vi "De Initialization.vi"(8 "Error In":errorcluster, 9 "Intialize?":bool=TRUE, 10 "Inputs":T1, 11 "Start SM":dbl=10.0 format="%#_13g") -> (0 "error out":errorcluster, 1 "Completed":bool, 3 "Results":cluster{"Pinch Force":dbl}, 4 "Status":cluster{"Status":string, "Elapsed Time":dbl}, 5 "Graph":dbl[][](array[numeric]))   [LabVIEW 2017]
doc: "Changelog:\n\n------------\nv0.1:\n- Bypass sensor 1 for all front\n\nv0.1:\n- Start Travel time taken from when the start moving command is given (previous state)\n- Total travel time is taken until the movement is stopped"
uses:
  controls/Model Name.ctl
  controls/All Inputs.ctl
  controls/SACB DI.ctl
  controls/De Intialization.ctl
  controls/FGV DO.ctl
panel:
  in  "Model Name":T3
  in  "minimum change 3":dbl=1.0 format="%#_13g"
  in  "minimum change 2":dbl=1.0 format="%#_13g"
  in  "minimum change":dbl=1.0 format="%#_13g"
  in  "AutoCommand":u32=30
  in  "Stall Time":u32=200
  out "Waveform Graph":dbl[][](graph)
  in  "Delay (for Rest)":u32=500
  in  "Timeout (ms)":u32=15000
  # "Inputs"
  # "Variables"
  # "Outputs"
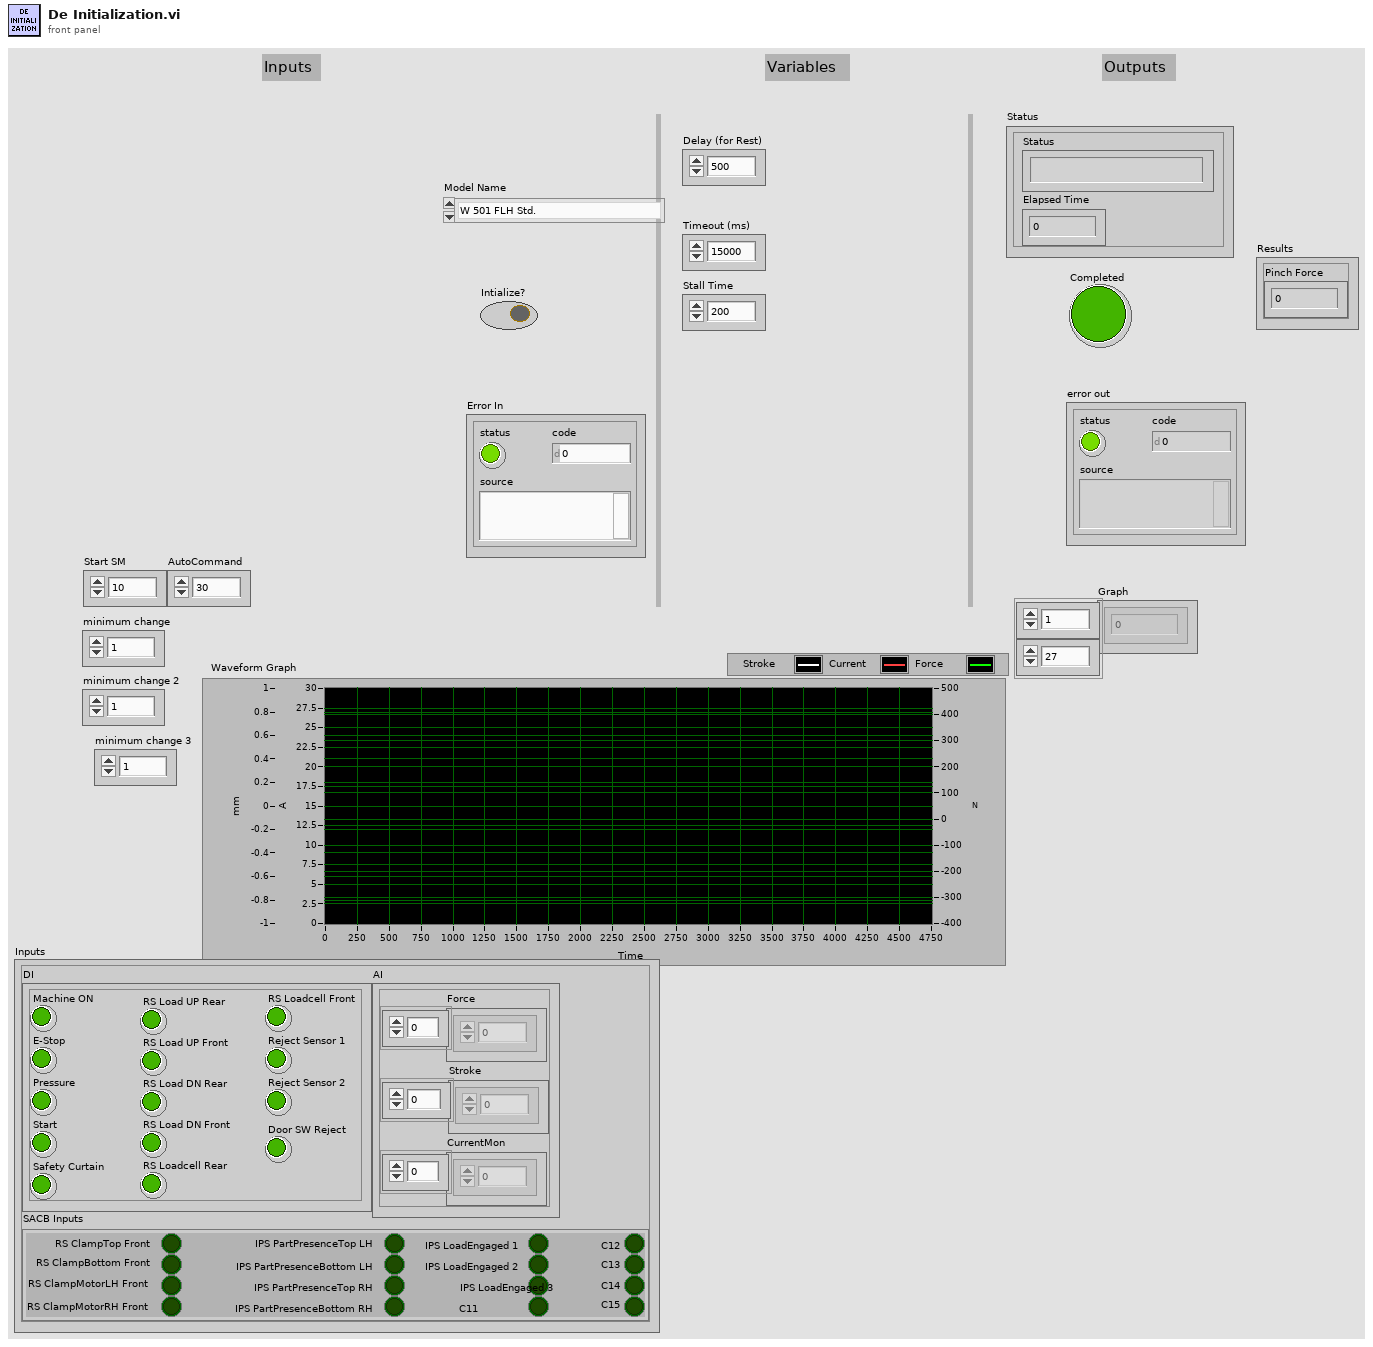
[diagram p1: front panel]
types:
  T1 = typedef "All Inputs.ctl" = cluster{"DI":cluster{"Machine ON":bool, "E-Stop":bool, "Pressure":bool, "Start":bool, "Safety Curtain":bool, "RS Load UP Rear":bool, "RS Load UP Front":bool, "RS Load DN Rear":bool, "RS Load DN Front":bool, "RS Loadcell Rear":bool, "RS Loadcell Front":bool, "Reject Sensor 1":bool, "Reject Sensor 2":bool, "Door SW Reject":bool}, "AI":cluster{"Force":dbl[], "Stroke":dbl[], "CurrentMon":dbl[]}, "SACB Inputs":T2}
  T2 = typedef "SACB DI.ctl" = cluster{"RS ClampTop Front":bool, "RS ClampBottom Front":bool, "RS ClampMotorLH Front":bool, "RS ClampMotorRH Front":bool, "IPS PartPresenceTop LH":bool, "IPS PartPresenceBottom LH":bool, "IPS PartPresenceTop RH":bool, "IPS PartPresenceBottom RH":bool, "IPS LoadEngaged 1":bool, "IPS LoadEngaged 2":bool, "IPS LoadEngaged 3":bool, "C11":bool, "C12":bool, "C13":bool, "C14":bool, "C15":bool}
  T3 = typedef "Model Name.ctl" = enum16{"W 501 FLH Std.", "W 501 FRH Std.", "W 601 FR RH Std", "W 601 FR LH Std", "W 601 RR RH Std", "W 601 RR LH Std", "W 601 FR RH AP", "W 601 FR LH AP", "W 601 RR RH AP", "W 601 RR LH AP"}
  T4 = typedef "De Intialization.ctl" = enum16{"Initialize", "Check Bottom Position", "Go Down", "Wait for Stall", "Go Up", "Wait for Top Stall", "Manual UP-1", "Manual UP-2", "Initialize Counter", "Auto UP-1", "Auto UP-2", "Wait for Stop", "Done", "Error"}
  T5 = typedef "FGV DO.ctl" = enum16{"Initialize", "Start Task", "Clamping", "Load CYL", "Contactors", "Loadcell CYL", "BSL", "Read DO", "Clear Tasks", "Clear Task"}
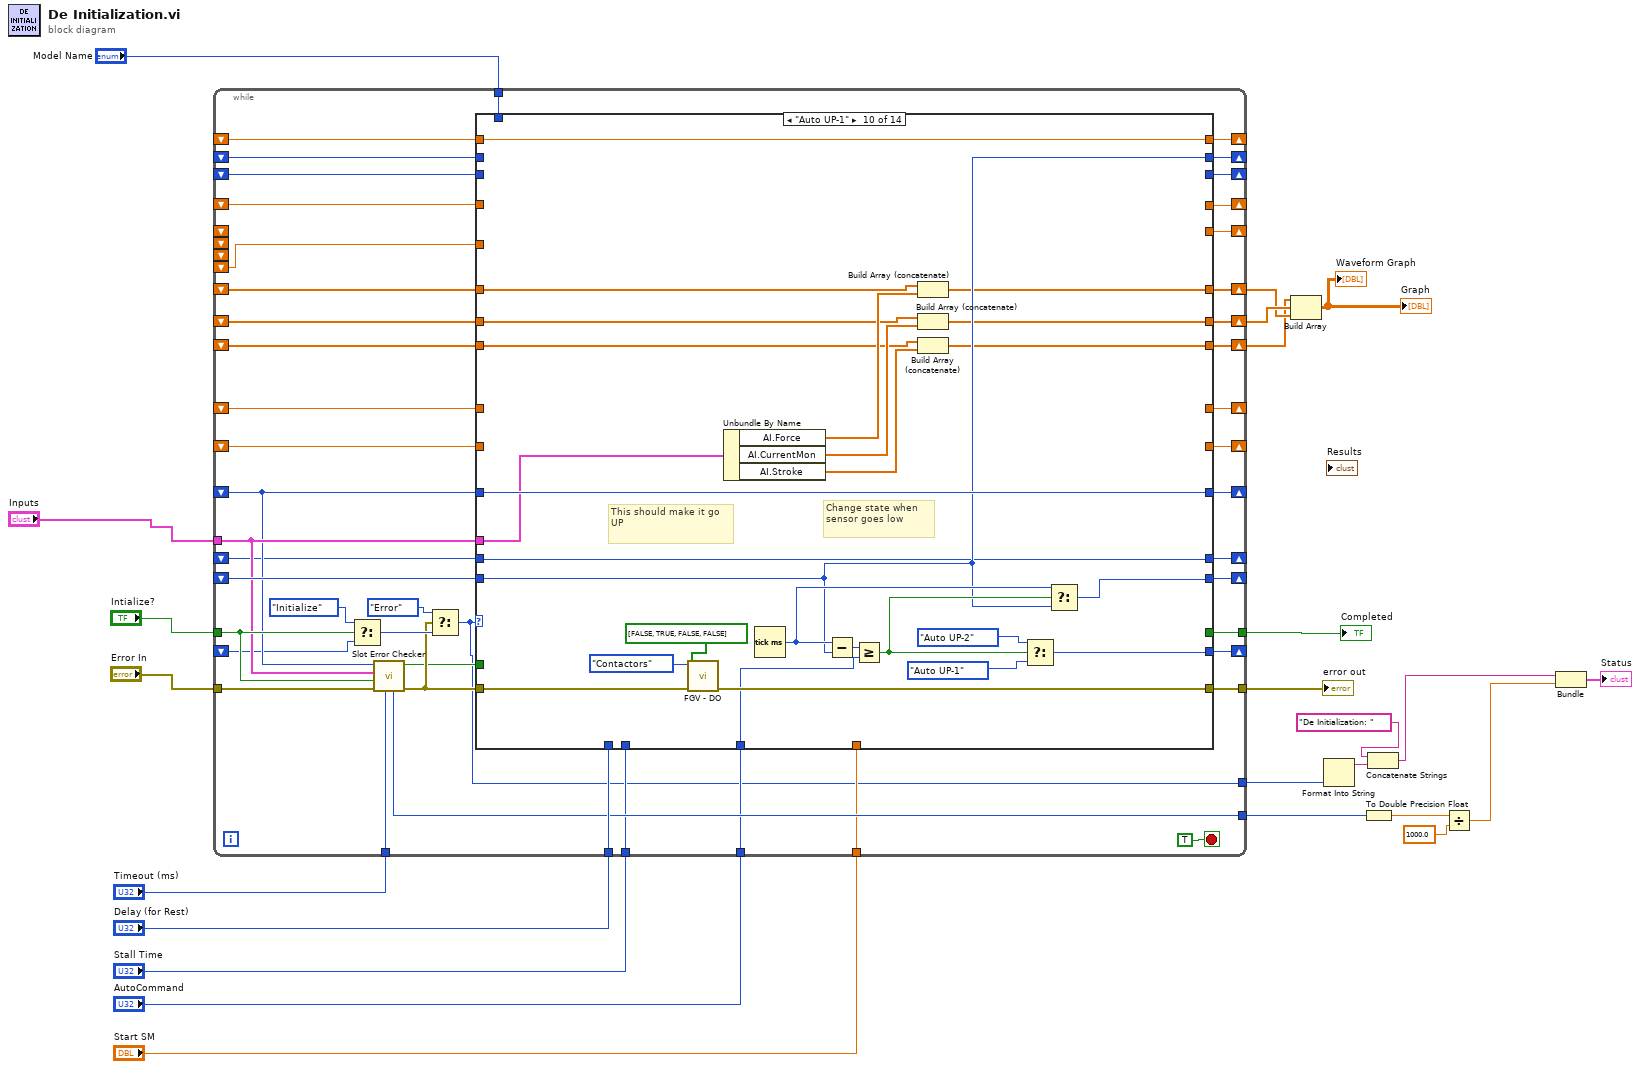
[diagram p0: block diagram]
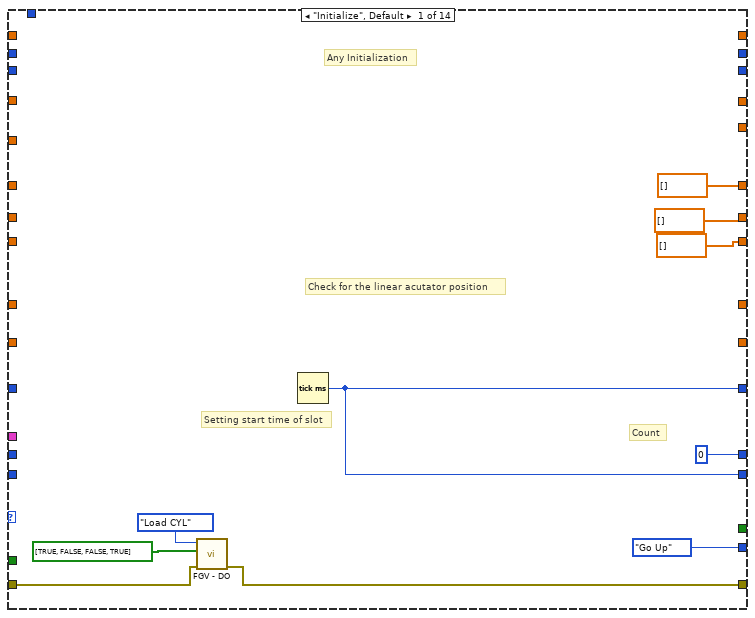
[diagram p2: hidden frame]
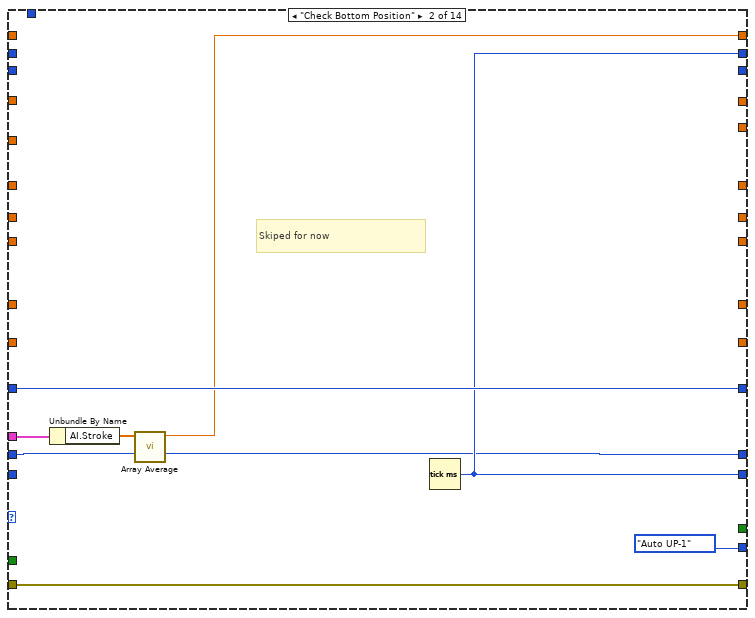
[diagram p3: hidden frame]
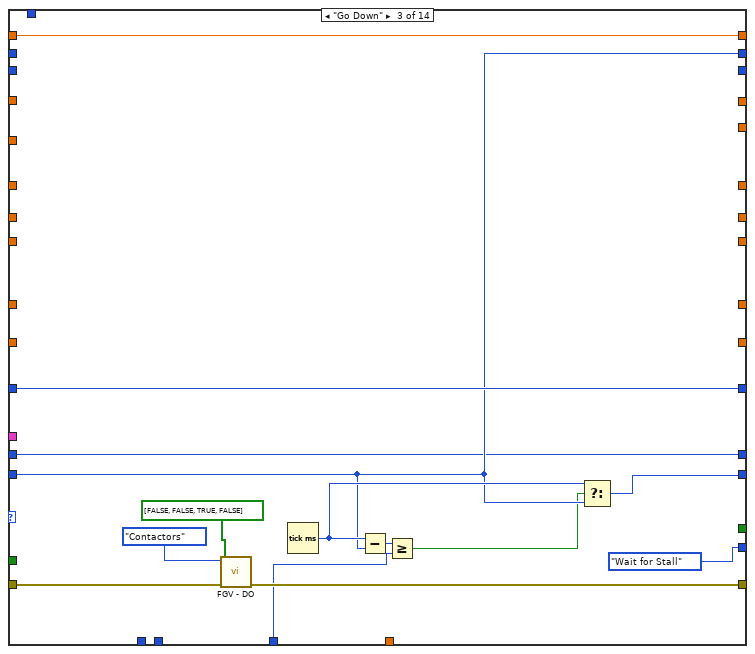
[diagram p4: hidden frame]
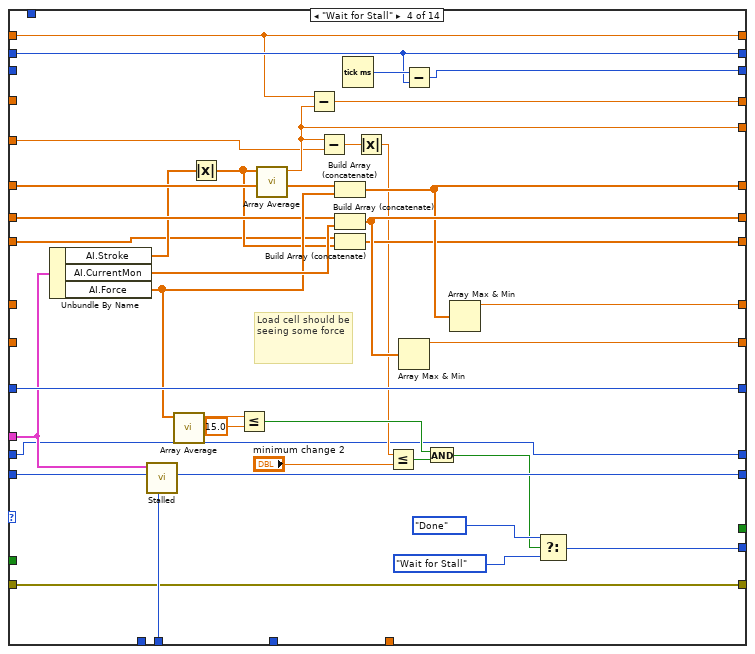
[diagram p5: hidden frame]
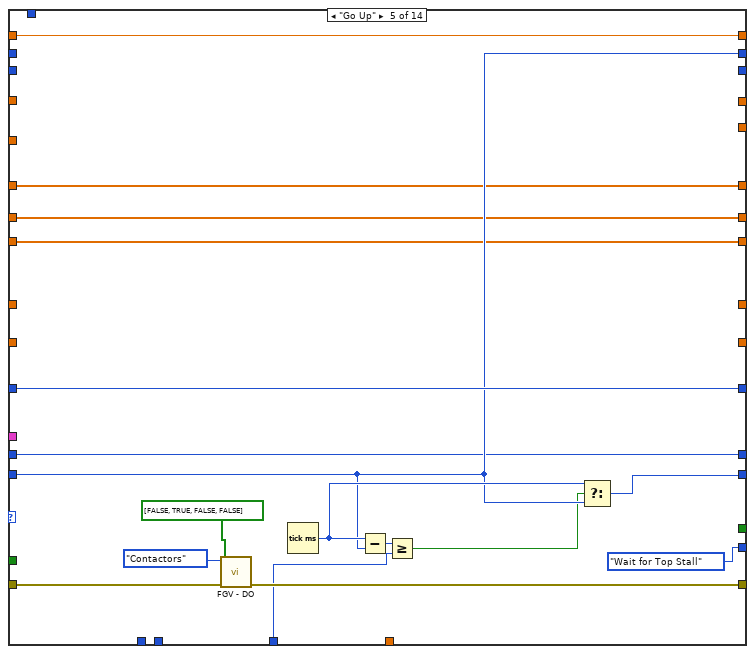
[diagram p6: hidden frame]
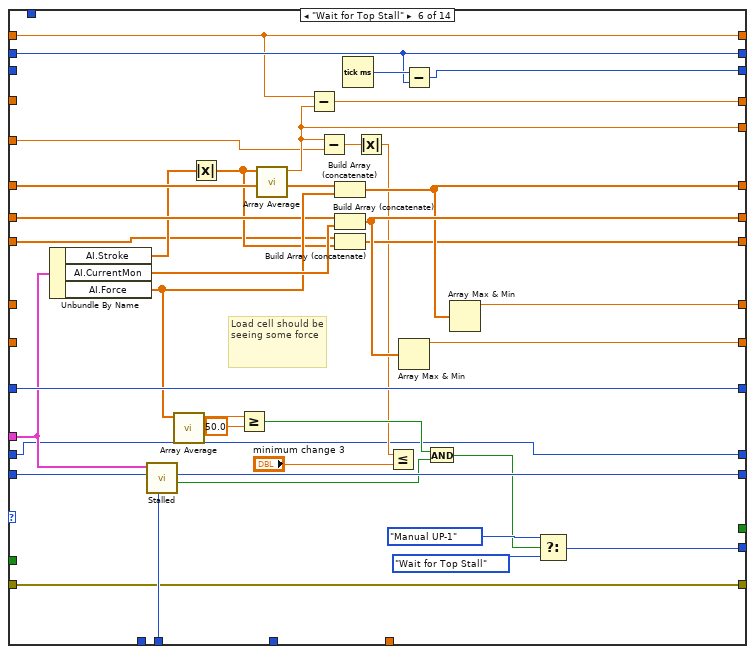
[diagram p7: hidden frame]
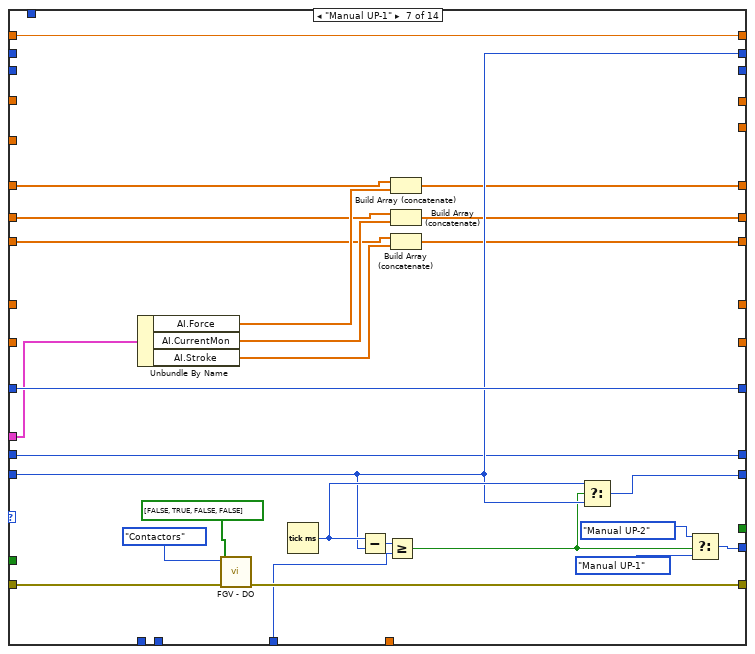
[diagram p8: hidden frame]
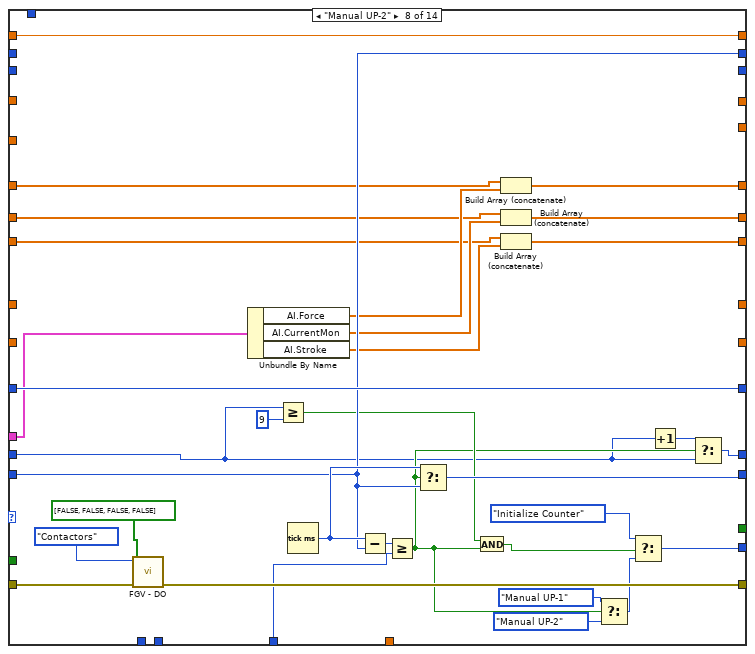
[diagram p9: hidden frame]
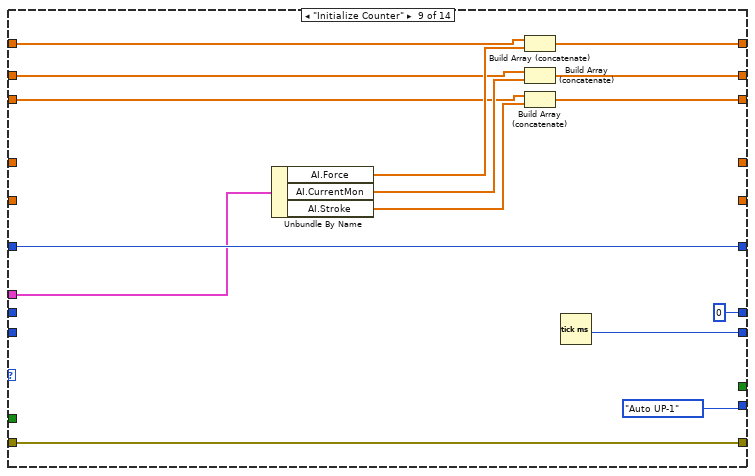
[diagram p10: hidden frame]
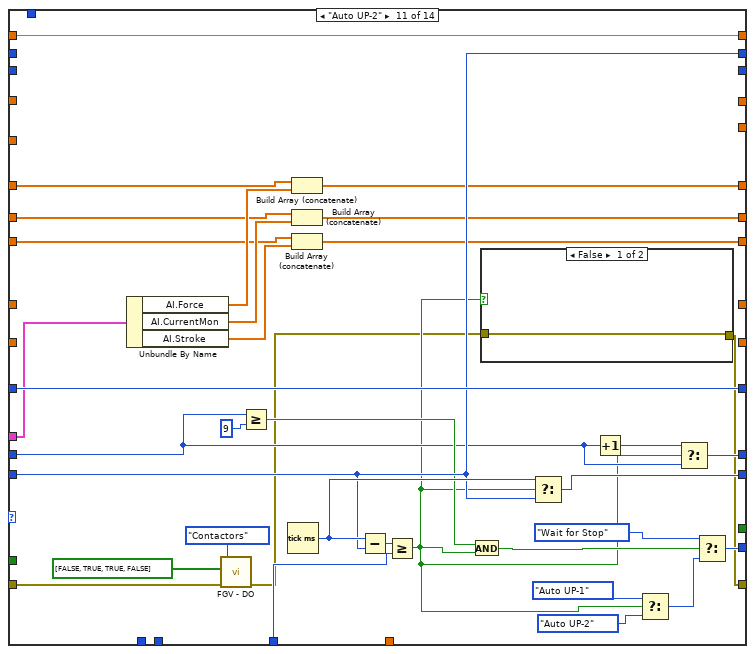
[diagram p11: hidden frame]
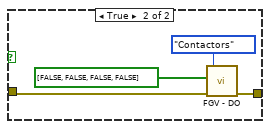
[diagram p12: hidden frame]
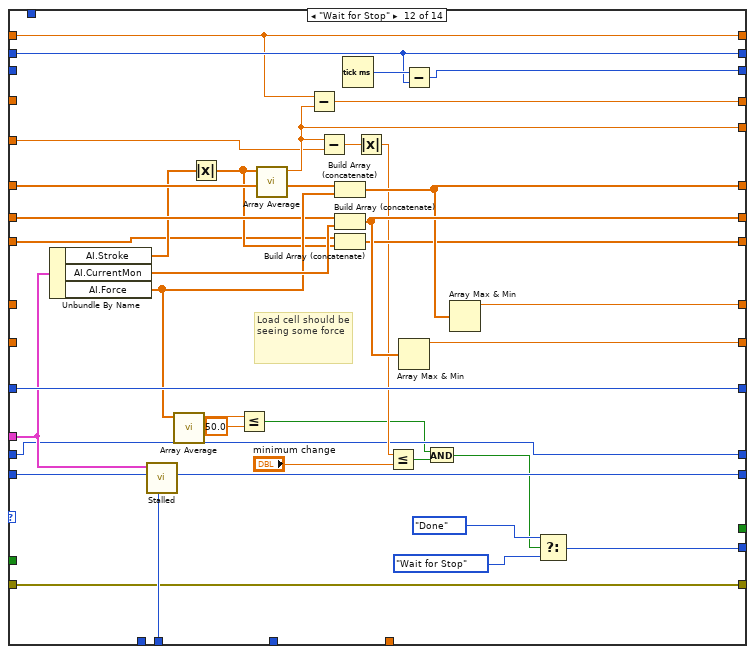
[diagram p13: hidden frame]
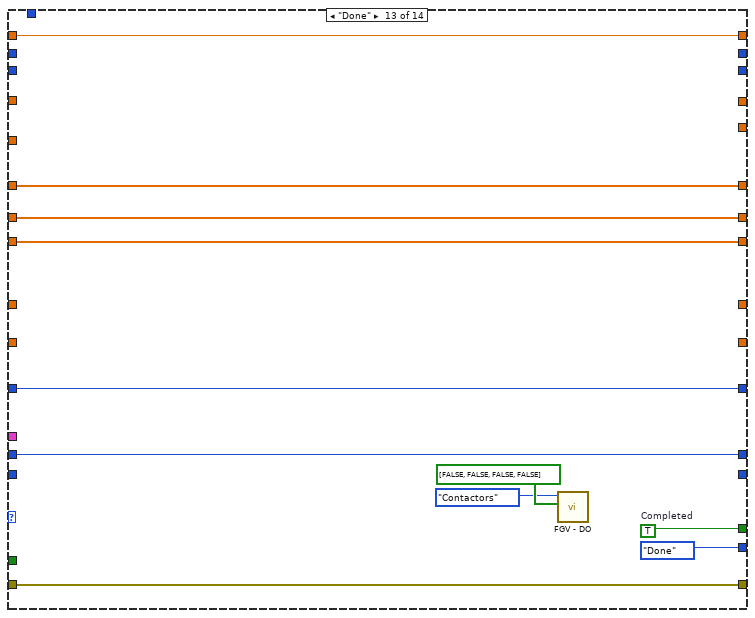
[diagram p14: hidden frame]
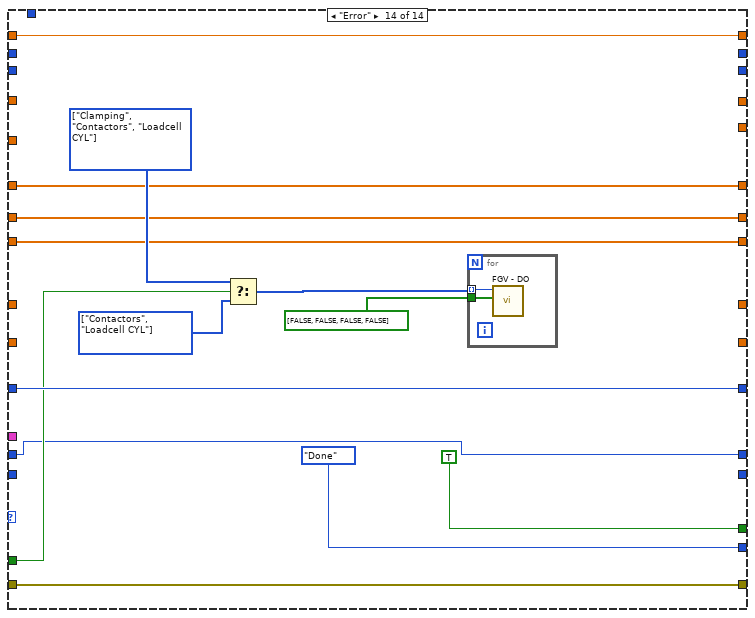
[diagram p15: hidden frame]
diagram:
  n1 = while {
    tunnel: "Intialize?" -> [w62]
    shift-right: [w69] -> _
    shift-left: _ -> [w26]
    shift-right: [w68] -> _
    shift-left: _ -> [w67]
    tunnel: "Error In" -> [w63]
    tunnel: [w66] -> w24
    tunnel: [w65] -> w23
    tunnel: "Inputs" -> [w61]
    shift-right: [w64] -> _
    shift-left: _ -> [w60]
    tunnel: "Delay (for Rest)" -> [w56]
    tunnel: "Timeout (ms)" -> [w55]
    tunnel: "Model Name" -> [w54]
    shift-right: [w53] -> _
    shift-left: _ -> [w52]
    shift-right: [w51] -> w7
    shift-left: _ -> [w50]
    shift-right: [w49] -> _
    shift-left: _ -> [w48]
    shift-right: [w47] -> _
    shift-left: _ -> [w46]
    tunnel: [w45] -> w14
    shift-right: [w44] -> _
    shift-left: _ -> [w43]
    shift-right: [w42] -> w13
    shift-left: _ -> [w41]
    shift-right: [w40] -> w11
    shift-left: _ -> [w39]
    shift-right: [w38] -> _
    shift-left: _ -> [w37]
    shift-right: [w36] -> _
    shift-left: _ -> [w35]
    tunnel: "Stall Time" -> [w34]
    tunnel: "Start SM" -> [w32]
    tunnel: "AutoCommand" -> [w31]
    shift-right: [w30] -> _
    shift-left: _ -> [_]
    shift-left: _ -> [_]
    shift-left: _ -> [_]
    shift-left: _ -> [w29]
    shift-right: [w28] -> _
    shift-left: _ -> [w27]
    tunnel: [w25] -> w1
    stop <- TRUE stop-if-true
    n2 = Select(t=De_Intialization."Initialize", s=w62, f=w26) -> (s? t:f=w59:T4)
    n3 = call "Slot Error Checker.vi"("Timeout (ms)"=w55, "error in (no error)"=w63, "Intialize?"=w62, "Inputs"=w61, "start time"=w60) -> ("error out"=w58:errorcluster, "Safety Interrupt?"=w33:bool, "Slot Time"=w45:u32)  [unwired: 4 in]
    n4 = Select(t=De_Intialization."Error", s=w58, f=w59) -> (s? t:f=w25:T4)
    n5 = case shown="\"Auto UP-1\"" w25 {
      tunnel: [De_Intialization."Go Up" De_Intialization."Auto UP-1" De_Intialization."Wait for Stall" w136 De_Intialization."Wait for Top Stall" w190 w213 w247 De_Intialization."Auto UP-1" w287 w322 w366 De_Intialization."Done" De_Intialization."Done"] -> w69
      tunnel: [w81 w83 w94 w127 w148 w181 w209 w243 w264 w282 w318 w357 _ _] -> w68
      tunnel: w67 -> [_ _ w95 w139 w149 w193 w210 w244 _ w283 w319 w369 _ _]
      tunnel: w58 -> [w78 w88 w93 w116 w147 w170 w207 w241 w265 w280 w328 w346 w380 w395]
      tunnel: [w77 w88 w103 w116 w157 w170 w220 w253 w265 w294 w305 w346 w380 w395] -> w66
      tunnel: [_ _ _ _ _ _ _ _ _ _ _ _ w379 TRUE ("Completed")] -> w65
      tunnel: w61 -> [_ w85 _ w105 _ w160 w204 w227 w254 w269 w295 w336 _ _]
      tunnel: [w81 w89 w101 w140 w155 w194 w218 w251 w267 w292 w326 w370 w378 w392] -> w64
      tunnel: w60 -> [_ w89 w101 w140 w155 w194 w218 w251 w267 w292 w326 w370 w378 w392]
      tunnel: w56 -> [_ _ _ _ _ _ _ _ _ _ _ _ _ _]
      tunnel: w54 -> [_ _ _ _ _ _ _ _ _ _ _ _ _ _]
      tunnel: [_ w83 w95 w126 w149 w180 w210 w244 _ w283 w319 w356 _ _] -> w53
      tunnel: w52 -> [_ _ _ w126 _ w180 _ _ _ _ _ w356 _ _]
      tunnel: [dbl[] [] _ _ w128 w141 w182 w196 w221 w257 w270 w296 w358 w377 w385] -> w51
      tunnel: w50 -> [_ _ _ w106 w141 w161 w197 w224 w258 w271 w297 w337 w377 w385]
      tunnel: [_ _ _ w129 _ w183 _ _ _ _ _ w359 _ _] -> w49
      tunnel: w48 -> [_ _ _ _ _ _ _ _ _ _ _ _ _ _]
      tunnel: [_ _ _ w134 _ w188 _ _ _ _ _ w364 _ _] -> w47
      tunnel: w46 -> [_ _ _ _ _ _ _ _ _ _ _ _ _ _]
      tunnel: [_ w84 w100 w117 w154 w171 w217 w250 _ w291 w325 w347 w375 w391] -> w44
      tunnel: w43 -> [_ _ w100 w117 w154 w171 w217 w250 _ w291 w325 w347 w375 w391]
      tunnel: [dbl[] [] _ _ w132 w142 w186 w199 w223 w256 w272 w298 w362 w376 w384] -> w42
      tunnel: w41 -> [_ _ _ w122 w142 w176 w200 w225 w259 w273 w299 w352 w376 w384]
      tunnel: [dbl[] [] _ _ w131 w143 w185 w201 w222 w255 w274 w300 w361 w372 w383] -> w40
      tunnel: w39 -> [_ _ _ w121 w143 w175 w202 w226 w260 w275 w301 w351 w372 w383]
      tunnel: [_ _ _ w130 _ w184 _ _ _ _ _ w360 _ _] -> w38
      tunnel: w37 -> [_ _ _ _ _ _ _ _ _ _ _ _ _ _]
      tunnel: [_ _ _ w114 _ w168 _ _ _ _ _ w345 _ _] -> w36
      tunnel: w35 -> [_ _ _ _ _ _ _ _ _ _ _ _ _ _]
      tunnel: w34 -> [_ _ _ w120 _ w174 _ _ _ _ _ w350 _ _]
      tunnel: w33 -> [_ _ _ _ _ _ _ _ _ _ _ _ _ w386]
      tunnel: w32 -> [_ _ _ _ _ _ _ _ _ _ _ _ _ _]
      tunnel: w31 -> [_ _ w97 _ w151 _ w212 w246 _ w286 w321 _ _ _]
      tunnel: [_ _ _ w113 _ w167 _ _ _ _ _ w344 _ _] -> w30
      tunnel: w29 -> [_ _ _ w112 _ w166 _ _ _ _ _ w343 _ _]
      tunnel: [0 w82 w91 w104 w145 w159 w205 w239 0 w279 w316 w335 w371 w382] -> w28
      tunnel: w27 -> [_ w82 w91 w104 w145 w159 w205 w231 _ w279 w308 w335 w371 w382]
      frame "Initialize", Default {
        # "Check for the linear acutator position"
        # "Count"
        # "Setting start time of slot"
        # "Any Initialization"
        n6 = call "FGV - DO.vi"("error in"=w78, "Digital Outs"=bool[] [TRUE, FALSE, FALSE, TRUE], "State"=FGV_DO."Load CYL") -> ("error out"=w77:errorcluster)  [unwired: 7 in, 1 out]
        n7 = Tick Count (ms)() -> (millisecond timer value=w81:u32)
      }
      frame "Check Bottom Position" {
        # "Skiped for now"
        n8 = Unbundle By Name(w85) -> ("AI.Stroke"=w86:dbl[])
        n9 = call "Array Average.vi"("data"=w86) -> ("Numeric"=w84:dbl)  [unwired: 10 in]
        n10 = Tick Count (ms)() -> (millisecond timer value=w83:u32)
      }
      frame "Go Down" {
        n11 = call "FGV - DO.vi"("error in"=w93, "Digital Outs"=bool[] [FALSE, FALSE, TRUE, FALSE], "State"=FGV_DO."Contactors") -> ("error out"=w103:errorcluster)  [unwired: 7 in, 1 out]
        n12 = Tick Count (ms)() -> (millisecond timer value=w96:u32)
        n13 = Subtract(x=w96, y=w95) -> (x-y=w98:u32)
        n14 = Greater Or Equal?(x=w98, y=w97) -> (x >= y?=w92:bool)
        n15 = Select(t=w96, s=w92, f=w95) -> (s? t:f=w94:u32)
      }
      frame "Wait for Stall" {
        # "Load cell should be seeing some force"
        n16 = Unbundle By Name(w105) -> ("AI.Stroke"=w119:dbl[], "AI.CurrentMon"=w133:dbl[], "AI.Force"=w124:dbl[])
        n17 = call "Stalled.vi"("Stall Time (ms)"=w120, "millisecond timer value in"=w139, "Inputs"=w105) -> ("millisecond timer value out"=w127:u32)  [unwired: 7 in, 1 out]
        n18 = call "Array Average.vi"("data"=w124) -> ("Numeric"=w123:dbl)  [unwired: 10 in]
        n19 = Absolute Value(x=w119) -> (abs(x)=w118:dbl[])
        n20 = Less Or Equal?(x=w123, y=15.0) -> (x <= y?=w115:bool)
        n21 = call "Array Average.vi"("data"=w118) -> ("Numeric"=w113:dbl)  [unwired: 10 in]
        n22 = Subtract(x=w117, y=w113) -> (x-y=w114:dbl)
        n23 = Subtract(x=w113, y=w112) -> (x-y=w111:dbl)
        n24 = Build Array (concatenate)(w121, w124) -> (w131:dbl[])
        n25 = Build Array (concatenate)(w122, w133) -> (w132:dbl[])
        n26 = Build Array (concatenate)(w106, w118) -> (w128:dbl[])
        n27 = Tick Count (ms)() -> (millisecond timer value=w135:u32)
        n28 = Absolute Value(x=w111) -> (abs(x)=w110:dbl)
        n29 = Less Or Equal?(x=w110, y="minimum change 2") -> (x <= y?=w107:bool)
        n30 = Array Max & Min(array=w132) -> (max value=w134:dbl)  [unwired: 3 out]
        n31 = Subtract(x=w135, y=w126) -> (x-y=w129:u32)
        n32 = And(x=w115, y=w107) -> (x .and. y?=w108:bool)
        n33 = Array Max & Min(array=w131) -> (max value=w130:dbl)  [unwired: 3 out]
        n34 = Select(t=De_Intialization."Done", s=w108, f=De_Intialization."Wait for Stall") -> (s? t:f=w136:T4)
      }
      frame "Go Up" {
        n35 = call "FGV - DO.vi"("error in"=w147, "Digital Outs"=bool[] [FALSE, TRUE, FALSE, FALSE], "State"=FGV_DO."Contactors") -> ("error out"=w157:errorcluster)  [unwired: 7 in, 1 out]
        n36 = Tick Count (ms)() -> (millisecond timer value=w150:u32)
        n37 = Subtract(x=w150, y=w149) -> (x-y=w152:u32)
        n38 = Greater Or Equal?(x=w152, y=w151) -> (x >= y?=w146:bool)
        n39 = Select(t=w150, s=w146, f=w149) -> (s? t:f=w148:u32)
      }
      frame "Wait for Top Stall" {
        # "Load cell should be seeing some force"
        n40 = Unbundle By Name(w160) -> ("AI.Stroke"=w173:dbl[], "AI.CurrentMon"=w187:dbl[], "AI.Force"=w178:dbl[])
        n41 = call "Stalled.vi"("Stall Time (ms)"=w174, "millisecond timer value in"=w193, "Inputs"=w160) -> ("Stalled"=w158:bool, "millisecond timer value out"=w181:u32)  [unwired: 7 in]
        n42 = call "Array Average.vi"("data"=w178) -> ("Numeric"=w177:dbl)  [unwired: 10 in]
        n43 = Absolute Value(x=w173) -> (abs(x)=w172:dbl[])
        n44 = Greater Or Equal?(x=w177, y=50.0) -> (x >= y?=w169:bool)
        n45 = call "Array Average.vi"("data"=w172) -> ("Numeric"=w167:dbl)  [unwired: 10 in]
        n46 = Subtract(x=w171, y=w167) -> (x-y=w168:dbl)
        n47 = Subtract(x=w167, y=w166) -> (x-y=w165:dbl)
        n48 = Build Array (concatenate)(w175, w178) -> (w185:dbl[])
        n49 = Build Array (concatenate)(w176, w187) -> (w186:dbl[])
        n50 = Build Array (concatenate)(w161, w172) -> (w182:dbl[])
        n51 = Tick Count (ms)() -> (millisecond timer value=w189:u32)
        n52 = Absolute Value(x=w165) -> (abs(x)=w164:dbl)
        n53 = Less Or Equal?(x=w164, y="minimum change 3") -> ()  [unwired: 1 out]
        n54 = Array Max & Min(array=w186) -> (max value=w188:dbl)  [unwired: 3 out]
        n55 = Subtract(x=w189, y=w180) -> (x-y=w183:u32)
        n56 = And(x=w169, y=w158) -> (x .and. y?=w162:bool)
        n57 = Array Max & Min(array=w185) -> (max value=w184:dbl)  [unwired: 3 out]
        n58 = Select(t=De_Intialization."Manual UP-1", s=w162, f=De_Intialization."Wait for Top Stall") -> (s? t:f=w190:T4)
      }
      frame "Manual UP-1" {
        n59 = Unbundle By Name(w204) -> ("AI.Force"=w203:dbl[], "AI.CurrentMon"=w198:dbl[], "AI.Stroke"=w195:dbl[])
        n60 = call "FGV - DO.vi"("error in"=w207, "Digital Outs"=bool[] [FALSE, TRUE, FALSE, FALSE], "State"=FGV_DO."Contactors") -> ("error out"=w220:errorcluster)  [unwired: 7 in, 1 out]
        n61 = Tick Count (ms)() -> (millisecond timer value=w211:u32)
        n62 = Subtract(x=w211, y=w210) -> (x-y=w215:u32)
        n63 = Greater Or Equal?(x=w215, y=w212) -> (x >= y?=w206:bool)
        n64 = Build Array (concatenate)(w202, w203) -> (w201:dbl[])
        n65 = Build Array (concatenate)(w200, w198) -> (w199:dbl[])
        n66 = Build Array (concatenate)(w197, w195) -> (w196:dbl[])
        n67 = Select(t=w211, s=w206, f=w210) -> (s? t:f=w209:u32)
        n68 = Select(t=De_Intialization."Manual UP-2", s=w206, f=De_Intialization."Manual UP-1") -> (s? t:f=w213:T4)
      }
      frame "Manual UP-2" {
        n69 = call "FGV - DO.vi"("error in"=w241, "Digital Outs"=bool[] [FALSE, FALSE, FALSE, FALSE], "State"=FGV_DO."Contactors") -> ("error out"=w253:errorcluster)  [unwired: 7 in, 1 out]
        n70 = Unbundle By Name(w227) -> ("AI.Force"=w230:dbl[], "AI.CurrentMon"=w229:dbl[], "AI.Stroke"=w228:dbl[])
        n71 = Greater Or Equal?(x=w231, y=9) -> (x >= y?=w237:bool)
        n72 = Tick Count (ms)() -> (millisecond timer value=w245:u32)
        n73 = Subtract(x=w245, y=w244) -> (x-y=w248:u32)
        n74 = Greater Or Equal?(x=w248, y=w246) -> (x >= y?=w233:bool)
        n75 = Select(t=w245, s=w233, f=w244) -> (s? t:f=w243:u32)
        n76 = And(x=w237, y=w233) -> (x .and. y?=w240:bool)
        n77 = Build Array (concatenate)(w226, w230) -> (w222:dbl[])
        n78 = Build Array (concatenate)(w225, w229) -> (w223:dbl[])
        n79 = Build Array (concatenate)(w224, w228) -> (w221:dbl[])
        n80 = Select(t=De_Intialization."Manual UP-1", s=w233, f=De_Intialization."Manual UP-2") -> (s? t:f=w234:T4)
        n81 = Select(t=De_Intialization."Initialize Counter", s=w240, f=w234) -> (s? t:f=w247:T4)
        n82 = Increment(x=w231) -> (x+1=w232:i32)
        n83 = Select(t=w232, s=w233, f=w231) -> (s? t:f=w239:i32)
      }
      frame "Initialize Counter" {
        n84 = Unbundle By Name(w254) -> ("AI.Force"=w263:dbl[], "AI.CurrentMon"=w262:dbl[], "AI.Stroke"=w261:dbl[])
        n85 = Build Array (concatenate)(w260, w263) -> (w255:dbl[])
        n86 = Build Array (concatenate)(w259, w262) -> (w256:dbl[])
        n87 = Build Array (concatenate)(w258, w261) -> (w257:dbl[])
        n88 = Tick Count (ms)() -> (millisecond timer value=w264:u32)
      }
      frame "Auto UP-1" {
        # "Change state when sensor goes low"
        # "This should make it go UP"
        n89 = call "FGV - DO.vi"("error in"=w280, "Digital Outs"=bool[] [FALSE, TRUE, FALSE, FALSE], "State"=FGV_DO."Contactors") -> ("error out"=w294:errorcluster)  [unwired: 7 in, 1 out]
        n90 = Unbundle By Name(w269) -> ("AI.Force"=w278:dbl[], "AI.CurrentMon"=w277:dbl[], "AI.Stroke"=w276:dbl[])
        n91 = Tick Count (ms)() -> (millisecond timer value=w284:u32)
        n92 = Subtract(x=w284, y=w283) -> (x-y=w289:u32)
        n93 = Greater Or Equal?(x=w289, y=w286) -> (x >= y?=w285:bool)
        n94 = Build Array (concatenate)(w275, w278) -> (w274:dbl[])
        n95 = Build Array (concatenate)(w273, w277) -> (w272:dbl[])
        n96 = Build Array (concatenate)(w271, w276) -> (w270:dbl[])
        n97 = Select(t=De_Intialization."Auto UP-2", s=w285, f=De_Intialization."Auto UP-1") -> (s? t:f=w287:T4)
        n98 = Select(t=w284, s=w285, f=w283) -> (s? t:f=w282:u32)
      }
      frame "Auto UP-2" {
        n99 = Unbundle By Name(w295) -> ("AI.Force"=w304:dbl[], "AI.CurrentMon"=w303:dbl[], "AI.Stroke"=w302:dbl[])
        n100 = call "FGV - DO.vi"("error in"=w328, "Digital Outs"=bool[] [FALSE, TRUE, TRUE, FALSE], "State"=FGV_DO."Contactors") -> ("error out"=w306:errorcluster)  [unwired: 7 in, 1 out]
        n101 = Greater Or Equal?(x=w308, y=9) -> (x >= y?=w314:bool)
        n102 = Tick Count (ms)() -> (millisecond timer value=w320:u32)
        n103 = Build Array (concatenate)(w301, w304) -> (w300:dbl[])
        n104 = Build Array (concatenate)(w299, w303) -> (w298:dbl[])
        n105 = Build Array (concatenate)(w297, w302) -> (w296:dbl[])
        n106 = Subtract(x=w320, y=w319) -> (x-y=w323:u32)
        n107 = Greater Or Equal?(x=w323, y=w321) -> (x >= y?=w307:bool)
        n108 = And(x=w314, y=w307) -> (x .and. y?=w313:bool)
        n109 = case shown="False" w307 {
          tunnel: w306 -> [w329 w331]
          tunnel: [w329 w330] -> w305
          frame False {
          }
          frame True {
            n110 = call "FGV - DO.vi"("error in"=w331, "Digital Outs"=bool[] [FALSE, FALSE, FALSE, FALSE], "State"=FGV_DO."Contactors") -> ("error out"=w330:errorcluster)  [unwired: 7 in, 1 out]
          }
        }
        n111 = Select(t=w320, s=w307, f=w319) -> (s? t:f=w318:u32)
        n112 = Increment(x=w308) -> (x+1=w309:i32)
        n113 = Select(t=De_Intialization."Auto UP-1", s=w307, f=De_Intialization."Auto UP-2") -> (s? t:f=w310:T4)
        n114 = Select(t=w309, s=w307, f=w308) -> (s? t:f=w316:i32)
        n115 = Select(t=De_Intialization."Wait for Stop", s=w313, f=w310) -> (s? t:f=w322:T4)
      }
      frame "Wait for Stop" {
        # "Load cell should be seeing some force"
        n116 = Unbundle By Name(w336) -> ("AI.Stroke"=w349:dbl[], "AI.CurrentMon"=w363:dbl[], "AI.Force"=w354:dbl[])
        n117 = call "Stalled.vi"("Stall Time (ms)"=w350, "millisecond timer value in"=w369, "Inputs"=w336) -> ("millisecond timer value out"=w357:u32)  [unwired: 7 in, 1 out]
        n118 = call "Array Average.vi"("data"=w354) -> ("Numeric"=w353:dbl)  [unwired: 10 in]
        n119 = Absolute Value(x=w349) -> (abs(x)=w348:dbl[])
        n120 = Less Or Equal?(x=w353, y=50.0) -> (x <= y?=w334:bool)
        n121 = call "Array Average.vi"("data"=w348) -> ("Numeric"=w344:dbl)  [unwired: 10 in]
        n122 = Subtract(x=w347, y=w344) -> (x-y=w345:dbl)
        n123 = Subtract(x=w344, y=w343) -> (x-y=w342:dbl)
        n124 = Build Array (concatenate)(w351, w354) -> (w361:dbl[])
        n125 = Build Array (concatenate)(w352, w363) -> (w362:dbl[])
        n126 = Build Array (concatenate)(w337, w348) -> (w358:dbl[])
        n127 = Tick Count (ms)() -> (millisecond timer value=w365:u32)
        n128 = Absolute Value(x=w342) -> (abs(x)=w341:dbl)
        n129 = Less Or Equal?(x=w341, y="minimum change") -> (x <= y?=w338:bool)
        n130 = Array Max & Min(array=w362) -> (max value=w364:dbl)  [unwired: 3 out]
        n131 = Subtract(x=w365, y=w356) -> (x-y=w359:u32)
        n132 = And(x=w334, y=w338) -> (x .and. y?=w339:bool)
        n133 = Array Max & Min(array=w361) -> (max value=w360:dbl)  [unwired: 3 out]
        n134 = Select(t=De_Intialization."Done", s=w339, f=De_Intialization."Wait for Stop") -> (s? t:f=w366:T4)
      }
      frame "Done" {
        w379 = TRUE  # Completed
        n135 = call "FGV - DO.vi"("Digital Outs"=bool[] [FALSE, FALSE, FALSE, FALSE], "State"=FGV_DO."Contactors") -> ()  [unwired: 8 in, 2 out]
      }
      frame "Error" {
        w387 = T5[] [enum."Contactors", enum."Loadcell CYL"] items=["Initialize", "Start Task", "Clamping", "Load CYL", "Contactors", "Loadcell CYL", "BSL", "Read DO", "Clear Tasks", "Clear Task"]
        w389 = T5[] [enum."Clamping", enum."Contactors", enum."Loadcell CYL"] items=["Initialize", "Start Task", "Clamping", "Load CYL", "Contactors", "Loadcell CYL", "BSL", "Read DO", "Clear Tasks", "Clear Task"]
        n136 = Select(t=w389, s=w386, f=w387) -> (s? t:f=w388:T5[])
        n137 = for {
          tunnel: w388 -> [w397] mode=indexing
          tunnel: bool[] [FALSE, FALSE, FALSE, FALSE] ("Digital Outs") -> [w396]
          n138 = call "FGV - DO.vi"("Digital Outs"=w396, "State"=w397) -> ()  [unwired: 8 in, 2 out]
        }
      }
    }
  }
  "error out" <- w24
  "Completed" <- w23
  n139 = Build Array(w7, w13, w11) -> (→"Graph" →"Waveform Graph":dbl[][])
  n140 = Format Into String(w1) -> (resulting string=w4:string)  [unwired: 3 in, 1 out]
  n141 = To Double Precision Float(number=w14) -> (double precision float=w18:dbl)
  n142 = Concatenate Strings("De Initialization: ", w4) -> (w2:string)
  n143 = Divide(x=w18, y=1000.0) -> (x/y=w16:dbl)
  n144 = Bundle(w2, w16) -> (→"Status":cluster{string, dbl})  [unwired: 1 in]
